vi "InstallVIPMPackage.vi"(8 "error in (no error)":errorcluster, 11 "VIPC File":path) -> (0 "error out":errorcluster)   [LabVIEW 2019]
uses:
  <vilib>/JKI/VIPM API/VIPM API_vipm_api.lvlib
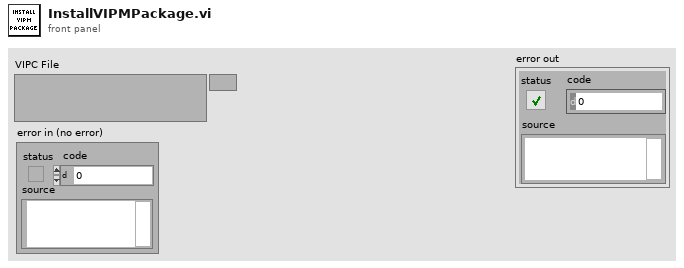
[diagram p1: front panel]
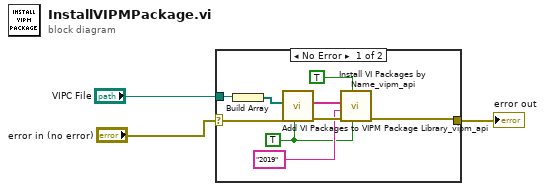
[diagram p0: block diagram]
diagram:
  n1 = case shown="No Error" "error in (no error)" {
    selector: "error in (no error)" -> [w10 w13]
    tunnel: [w4 w13] -> w2
    tunnel: "VIPC File" -> [w12 _]
    frame No Error {
      w5 = TRUE ("quiet? (T)")
      n2 = Build Array(w12) -> (w11:path[])
      n3 = call <vilib>:"Add VI Packages to VIPM Package Library_vipm_api.vi"("quiet? (T)"=w5, "error in (no error)"=w10, "Packages to add to VIPM Library (vipc,vip,ogp)"=w11) -> ("error out"=w9:errorcluster, "Package Names Added"=w8:string[])  [unwired: 7 in]
      n4 = call <vilib>:"Install VI Packages by Name_vipm_api.vi"("quiet? (T)"=w5, "accept-eulas? (T)"=TRUE, "error in (no error)"=w9, "LabVIEW Version"="2019", "Package Names to Install []"=w8) -> ("error out"=w4:errorcluster)  [unwired: 6 in]
    }
    frame Error {
    }
  }
  "error out" <- w2
